vi "Gyro Start I2C.vi"(8 "error in":errorcluster, 11 "FPGA Reference In":T1) -> (0 "error out":errorcluster, 3 "I2C Information Out":T2)   [LabVIEW 2012]
uses:
  FPGA_ref.ctl
  <vilib>/IEDriver/SPIandI2C/Host/I2C/I2C Host.lvlib
panel:
  in  "Clock Rate":u32=5000
  in  "Address Type (7-bit)":enum16{"7-bit", "10-bit"}(ring)
  in  "Address":u16=104 format="%.0x"
  in  "FPGA Clock (40 MHz)":u32=40000000
  in  "Port Number":u8
  # "I2C GYRO CONFIG\n-----------------------\nMust be called eacht ime to setup I2C transfer\nto ITG3505 Gyro"
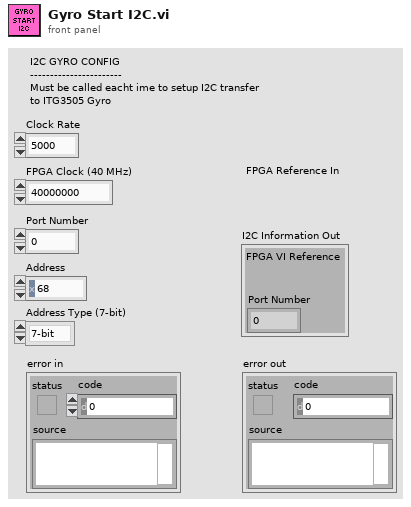
[diagram p1: front panel]
types:
  T1 = typedef "FPGA_ref.ctl" = refnum<k20>
  T2 = cluster{"FPGA VI Reference":refnum<k20>, "Port Number":u8}
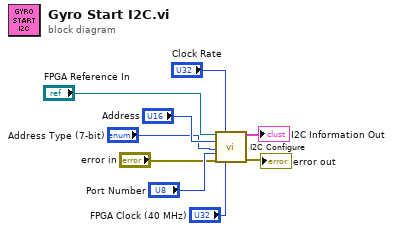
[diagram p0: block diagram]
diagram:
  n1 = call <vilib>:"I2C Configure.vi"("FPGA VI Reference"="FPGA Reference In", "Clock Rate"="Clock Rate", "Address"="Address", "Address Type (7-bit)"="Address Type (7-bit)", "Port Number"="Port Number", "error in (no error)"="error in", "FPGA Clock (40 MHz)"="FPGA Clock (40 MHz)") -> ("FPGA Information Out"=→"I2C Information Out":T2, "error out"=→"error out":errorcluster)  [unwired: 7 in]
